vi "Handle Notification.vi"(8 "error in (no error)":errorcluster, 9 "Payload":string, 10 "Notification Type":string, 11 "Analog Tachometer in":refnum<class "Analog Tachometer Process.lvclass">) -> (0 "error out":errorcluster, 3 "Analog Tachometer out":refnum<class "Analog Tachometer Process.lvclass">)   [LabVIEW 2024, in "Analog Tachometer Process.lvlib" / "Analog Tachometer Process.lvclass"]
uses:
  Analog Tachometer Process.lvclass
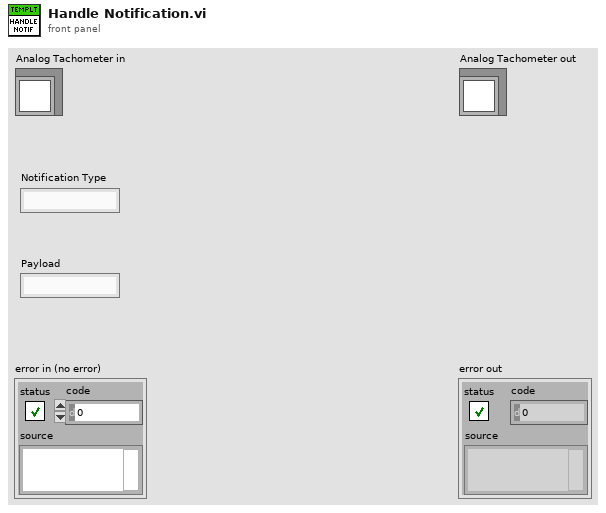
[diagram p1: front panel]
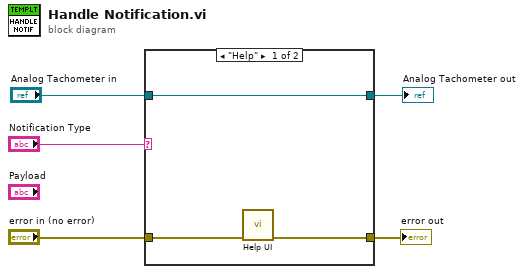
[diagram p0: block diagram]
diagram:
  n1 = case shown="\"Help\"" "Notification Type" {
    tunnel: "Analog Tachometer in" -> [w8 w10]
    tunnel: [w8 w10] -> w3
    tunnel: [w6 w9] -> w2
    tunnel: "error in (no error)" -> [w7 w9]
    frame "Help" {
      n2 = call "Help UI.vi"("error in (no error)"=w7) -> ("error out"=w6:errorcluster)  [unwired: 10 in]
    }
    frame Default {
    }
  }
  "error out" <- w2
  "Analog Tachometer out" <- w3
